vi "load data.vi"(8 "error in":errorcluster, 10 "file name":string) -> (0 "error out":errorcluster, 2 "Data Array":string[](array[string]))   [LabVIEW 2021]
panel:
  out "appended path":path
  out "file path (out)":path
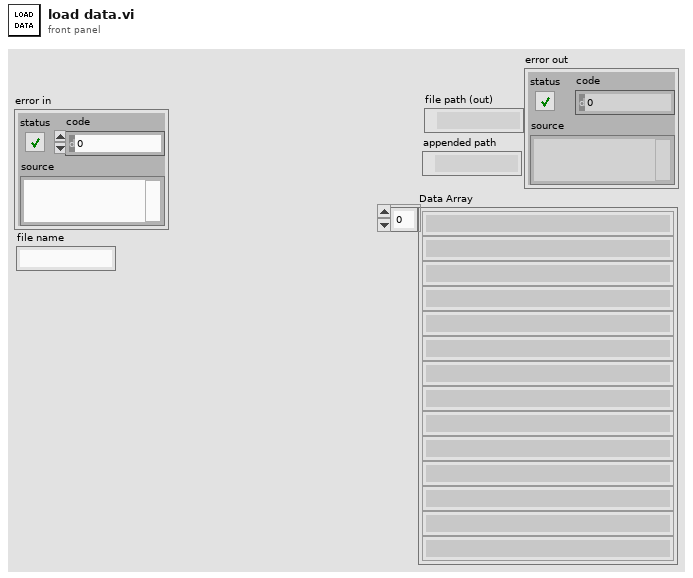
[diagram p1: front panel]
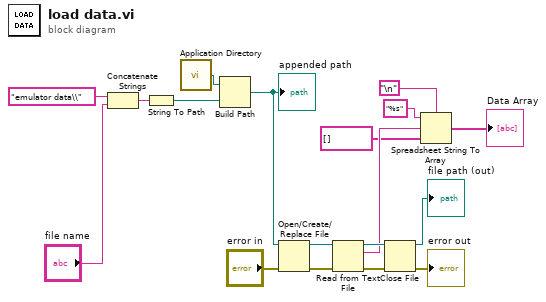
[diagram p0: block diagram]
diagram:
  n1 = Concatenate Strings("emulator data\\" ("string"), "file name") -> (w7:string)
  n2 = String To Path(string=w7) -> (path=w9:path)
  n3 = call <vilib>:"Application Directory.vi"() -> ("Application Directory"=w11:path)
  n4 = Build Path(base path=w11, name or relative path=w9) -> (appended path=w8:path)
  "appended path" <- w8
  n5 = Open/Create/Replace File(file path (use dialog)=w8, error in="error in") -> (refnum out=w18:refnum<file>, error out=w15:errorcluster)  [unwired: 4 in, 1 out]
  n6 = Read from Text File(file (use dialog)=w18, error in=w15) -> (refnum out=w17:refnum<file>, text=w4:string, error out=w14:errorcluster)  [unwired: 2 in, 1 out]
  n7 = Close File(refnum=w17, error in=w14) -> (path=→"file path (out)":path, error out=→"error out":errorcluster)
  n8 = Spreadsheet String To Array(delimiter (Tab)="\n", format string="%s", spreadsheet string=w4, array type (2D Dbl)=string[] []) -> (array=→"Data Array":string[])
